vi "WF phase diversity_MATLAB_Correction_loop_AndorSDK_CorrForEachZ.vi"() -> ()   [LabVIEW 2018]
uses:
  <userlib>/WaveKit.lib/Controls/Wavefront Corrector states - ONE.ctl
  <userlib>/WaveKit.lib/Classes/WavefrontCorrector/WavefrontCorrector.lvclass
  <userlib>/WaveKit.lib/Classes/WavefrontCorrectorSet/WavefrontCorrectorSet.lvclass
  <vilib>/Analysis/1siggen.llb/Ramp Pattern by Samples.vi
  <vilib>/Utility/file.llb/Read From Spreadsheet File (DBL).vi
  <vilib>/Analysis/1siggen.llb/Ramp Pattern by Delta.vi
  <vilib>/Analysis/NI_AALBase.lvlib
panel:
  in  "Tab Control":T1(tab)
  in  "Offset command file":path=path "D:/SystemAlignment/system_aberration_20200206.dat"
  in  "Initial haso file":path=path "D:/SystemAlignment/system_aberration_residual_20191015.has"
  out "# of Phase":i32
  in  "Error in":errorcluster
  in  "DM configuration file":path=path "C:/Program Files (x86)/Imagine Optic/Configuration Files/WaveFrontCorrector_mirao52-e_0326.dat"
  out "DM Initial State":T2[](array[typedef])
  out "DM ActuatorsNumber":i32
  out "Error out":errorcluster
  in  "EMCCD trigger port":tag="Dev1/port0/line0"
  in  "Cooler set to Temperature":i32=-60
  in  "Trigger":u32(ring)=1 items=["Internal", "External"]
  out "Return from CheckTimings":u32
  out "Calculated Exposure Value":sgl format="%.2f"
  out "Return from SetTemperature":u32
  out "Cooling":i32
  out "Return from Initialize":u32
  out "Detector X Pixels":i32
  out "Detector Y Pixels":i32
  in  "Initialize EMCCD?":bool=TRUE
  in  "Turn off EMCCD when finished?":bool=TRUE
  in  "Initial Zer coeff":dbl[](array[numeric])=[0.2, 0.2]
  in  "Initial Zer index":dbl[](array[numeric])=[4.0, 5.0]
  out "Initial Zer coeff\nRandomly generated":dbl[](array[numeric])
  out "Initial Zer index (starting from 4)\nrandomly generated":dbl[](array[numeric])
  in  "aberration tolerance":dbl=0.1 format="%#_13g"
  in  "aberration threshold":dbl=0.25 format="%#_13g"
  in  "?":enum16{"input manually ", "randomly generated"}(ring)
  in  "max random order":i64=9
  in  "NOT YET: Data Acquisition Iteration #":i32=1
  in  "Zern index in 2":i32[](array[numeric])=[3, 4, 5, 6, 7, 8]
  in  "Zern coef in 2":sgl[](array[numeric])=[0.0, 0.0, 0.2, 0.0, 0.0, 0.0]
  in  "Zern index in 3":i32[](array[numeric])=[3, 4, 5, 6, 7, 8]
  in  "Zern coef in 3":sgl[](array[numeric])=[0.2, 0.0, 0.0, 0.0, 0.0, 0.0]
  in  "Zern index in 4":i32[](array[numeric])=[3, 4, 5, 6, 7, 8]
  in  "Zern coef in 4":sgl[](array[numeric])=[0.2, 0.0, 0.0, 0.0, 0.0, 0.0]
  in  "Zern index in 5":i32[](array[numeric])=[3, 4, 5, 6, 7, 8]
  in  "Zern coef in 5":sgl[](array[numeric])=[0.0, 0.0, 0.0, 0.0, 0.0, -0.2]
  in  "Andor Picture/notes save to path":path=path "D:/YD/test/test1"
  in  "base name":string="beads_test"
  in  "Pics/phase":dbl=2.0
  in  "camera exposure time (s)":string="0.02"
  in  "# of Phase":i32=5
  in  "COMMAND matrix path":path=path "D:/SystemAlignment/IM_20200224.aomi"
  in  "488 shutter":refnum<k7>(container)
  in  "?":bool
  out "phase diversity file name":string
  out "Corrected Picture name":string
  in  "Z scanning range (um)":dbl format="%#_13g"
  in  "Z scanning step (um)":dbl format="%#_13g"
  in  "center Z (um) (10 steps=1um)":dbl format="%#_13g"
  in  "ASI stage VISA resource name":refnum<visa-resource-name>="COM5"
  out "current z step (10 steps=1um)":string="where z"
  in  "Use GPU":bool=TRUE
  in  "Show Recon":bool=TRUE
  in  "Show Input":bool
  in  "Background Value":u32=290
  in  "Crop Size of image":u32=512
  in  "Gamma Value":dbl=1e-06
  in  "Iteration Number":u32=10
  in  "Zernike Order":u32=15
  in  "Number for average":u32=2
  in  "Number of Phase":u32=2
  in  "Run MATLAB or correction?":bool=TRUE
  in  "Keep Reconstructed Defocus component?":bool
  # "Cooler is off for testing"
  # "If Pics/phase is 2:\npicture order:\n\noffset+aberr *2\nphase diversity *8\n\nground truth *1\noffset+aberr *1\ncorrected *2 but the last one cannot be seen in imagej"
  # "Randomly Generate Initial Zernike, enter here:"
  # "Manually input, enter here:"
  # "Andor Camera Settings"
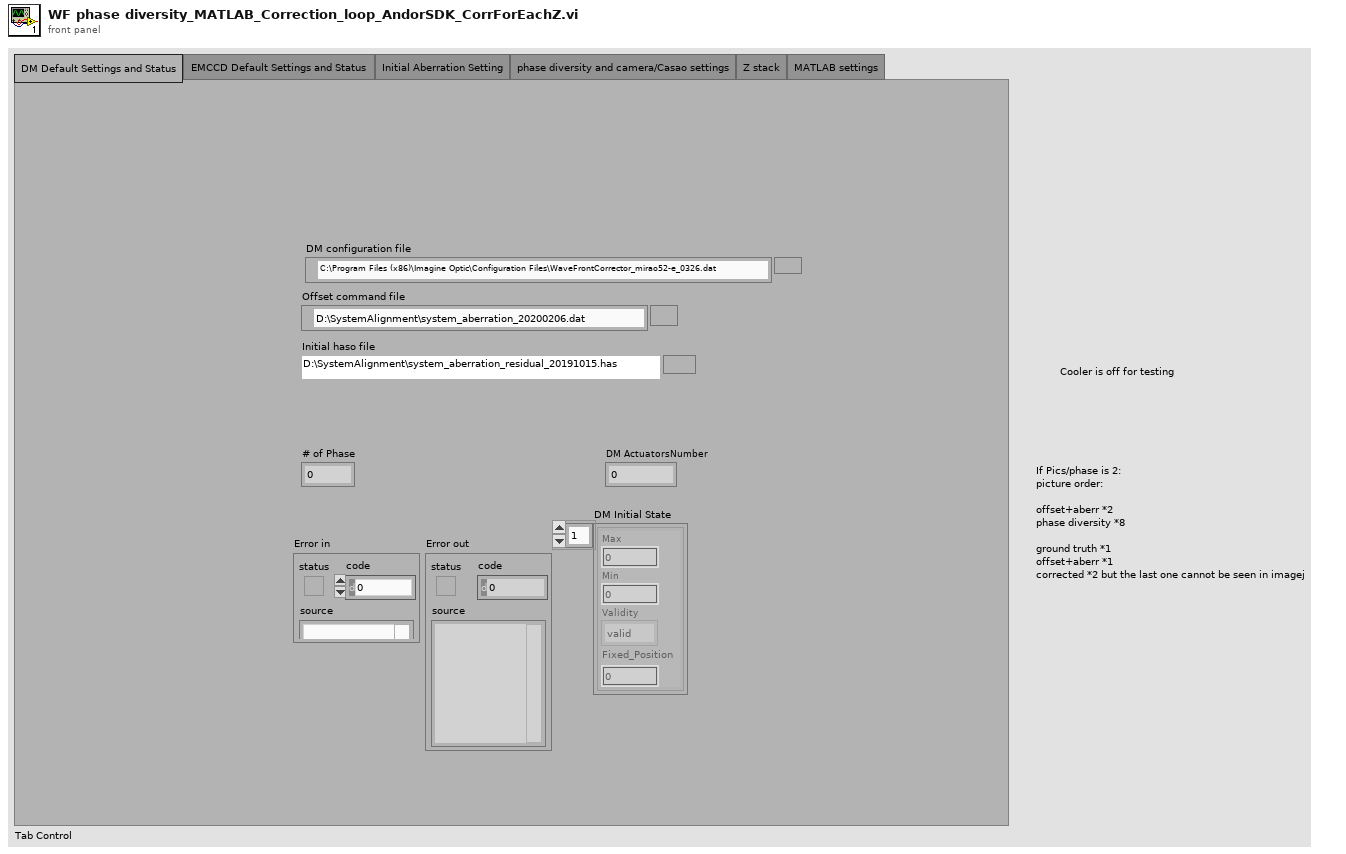
[diagram p1: front panel]
types:
  T1 = enum32{"DM Default Settings and Status", "EMCCD Default Settings and Status ", "Initial Aberration Setting", "phase diversity and camera/Casao settings", "Z stack", "MATLAB settings"}
  T2 = typedef "Wavefront Corrector states - ONE.ctl" = cluster{"Max":sgl, "Min":sgl, "Validity":enum16{"valid", "fixed", "invalid"}, "Fixed_Position":sgl}
  T3 = typedef "Error Code Enum typedef.ctl" = enum32{"N/A (0)", "DRV_ERROR_CODES", "DRV_SUCCESS", "DRV_VXDNOTINSTALLED", "DRV_ERROR_SCAN", "DRV_ERROR_CHECK_SUM", "DRV_ERROR_FILELOAD", "DRV_UNKNOWN_FUNC", "DRV_ERROR_VXD_INIT", "DRV_ERROR_ADDRESS", "DRV_ERROR_PAGELOCK", "DRV_ERROR_PAGEUNLOCK", "DRV_ERROR_BOARDTEST", "DRV_ERROR_ACK", "DRV_ERROR_UP_FIFO", "DRV_ERROR_PATTERN", "N/A (16)", "DRV_ACQUISITION_ERRORS", "DRV_ACQ_BUFFER", "DRV_ACQ_DOWNFIFO_FULL", "DRV_PROC_UNKONWN_INSTRUCTION", "DRV_ILLEGAL_OP_CODE", "DRV_KINETIC_TIME_NOT_MET", "DRV_ACCUM_TIME_NOT_MET", "DRV_NO_NEW_DATA", "N/A (25)", "DRV_SPOOLERROR", "N/A (27)", "N/A (28)", "N/A (29)", "N/A (30)", "N/A (31)", "N/A (32)", "DRV_TEMPERATURE_CODES", "DRV_TEMPERATURE_OFF", "DRV_TEMPERATURE_NOT_STABILIZED", "DRV_TEMPERATURE_STABILIZED", "DRV_TEMPERATURE_NOT_REACHED", "DRV_TEMPERATURE_OUT_RANGE", "DRV_TEMPERATURE_NOT_SUPPORTED", "DRV_TEMPERATURE_DRIFT", "N/A (41)", "N/A (42)", "N/A (43)", "N/A (44)", "N/A (45)", "N/A (46)", "N/A (47)", "N/A (48)", "DRV_GENERAL_ERRORS", "DRV_INVALID_AUX", "DRV_COF_NOTLOADED", "DRV_FPGAPROG", "DRV_FLEXERROR", "DRV_GPIBERROR", "N/A (55)", "N/A (56)", "N/A (57)", "N/A (58)", "N/A (59)", "N/A (60)", "N/A (61)", "N/A (62)", "N/A (63)", "DRV_DATATYPE", "DRV_DRIVER_ERRORS", "DRV_P1INVALID", "DRV_P2INVALID", "DRV_P3INVALID", "DRV_P4INVALID", "DRV_INIERROR", "DRV_COFERROR", "DRV_ACQUIRING", "DRV_IDLE", "DRV_TEMPCYCLE", "DRV_NOT_INITIALIZED", "DRV_P5INVALID", "DRV_P6INVALID", "DRV_INVALID_MODE", "DRV_INVALID_FILTER", "DRV_I2CERRORS", "DRV_I2CDEVNOTFOUND", "DRV_I2CTIMEOUT", "DRV_P7INVALID", "N/A (84)", "N/A (85)", "N/A (86)", "N/A (87)", "N/A (88)", "N/A (89)", "DRV_IOCERROR", "DRV_VRMVERSIONERROR"}
  T4 = typedef "NI_Matrix.lvlib/RealMatrix.ctl" = dbl[][]
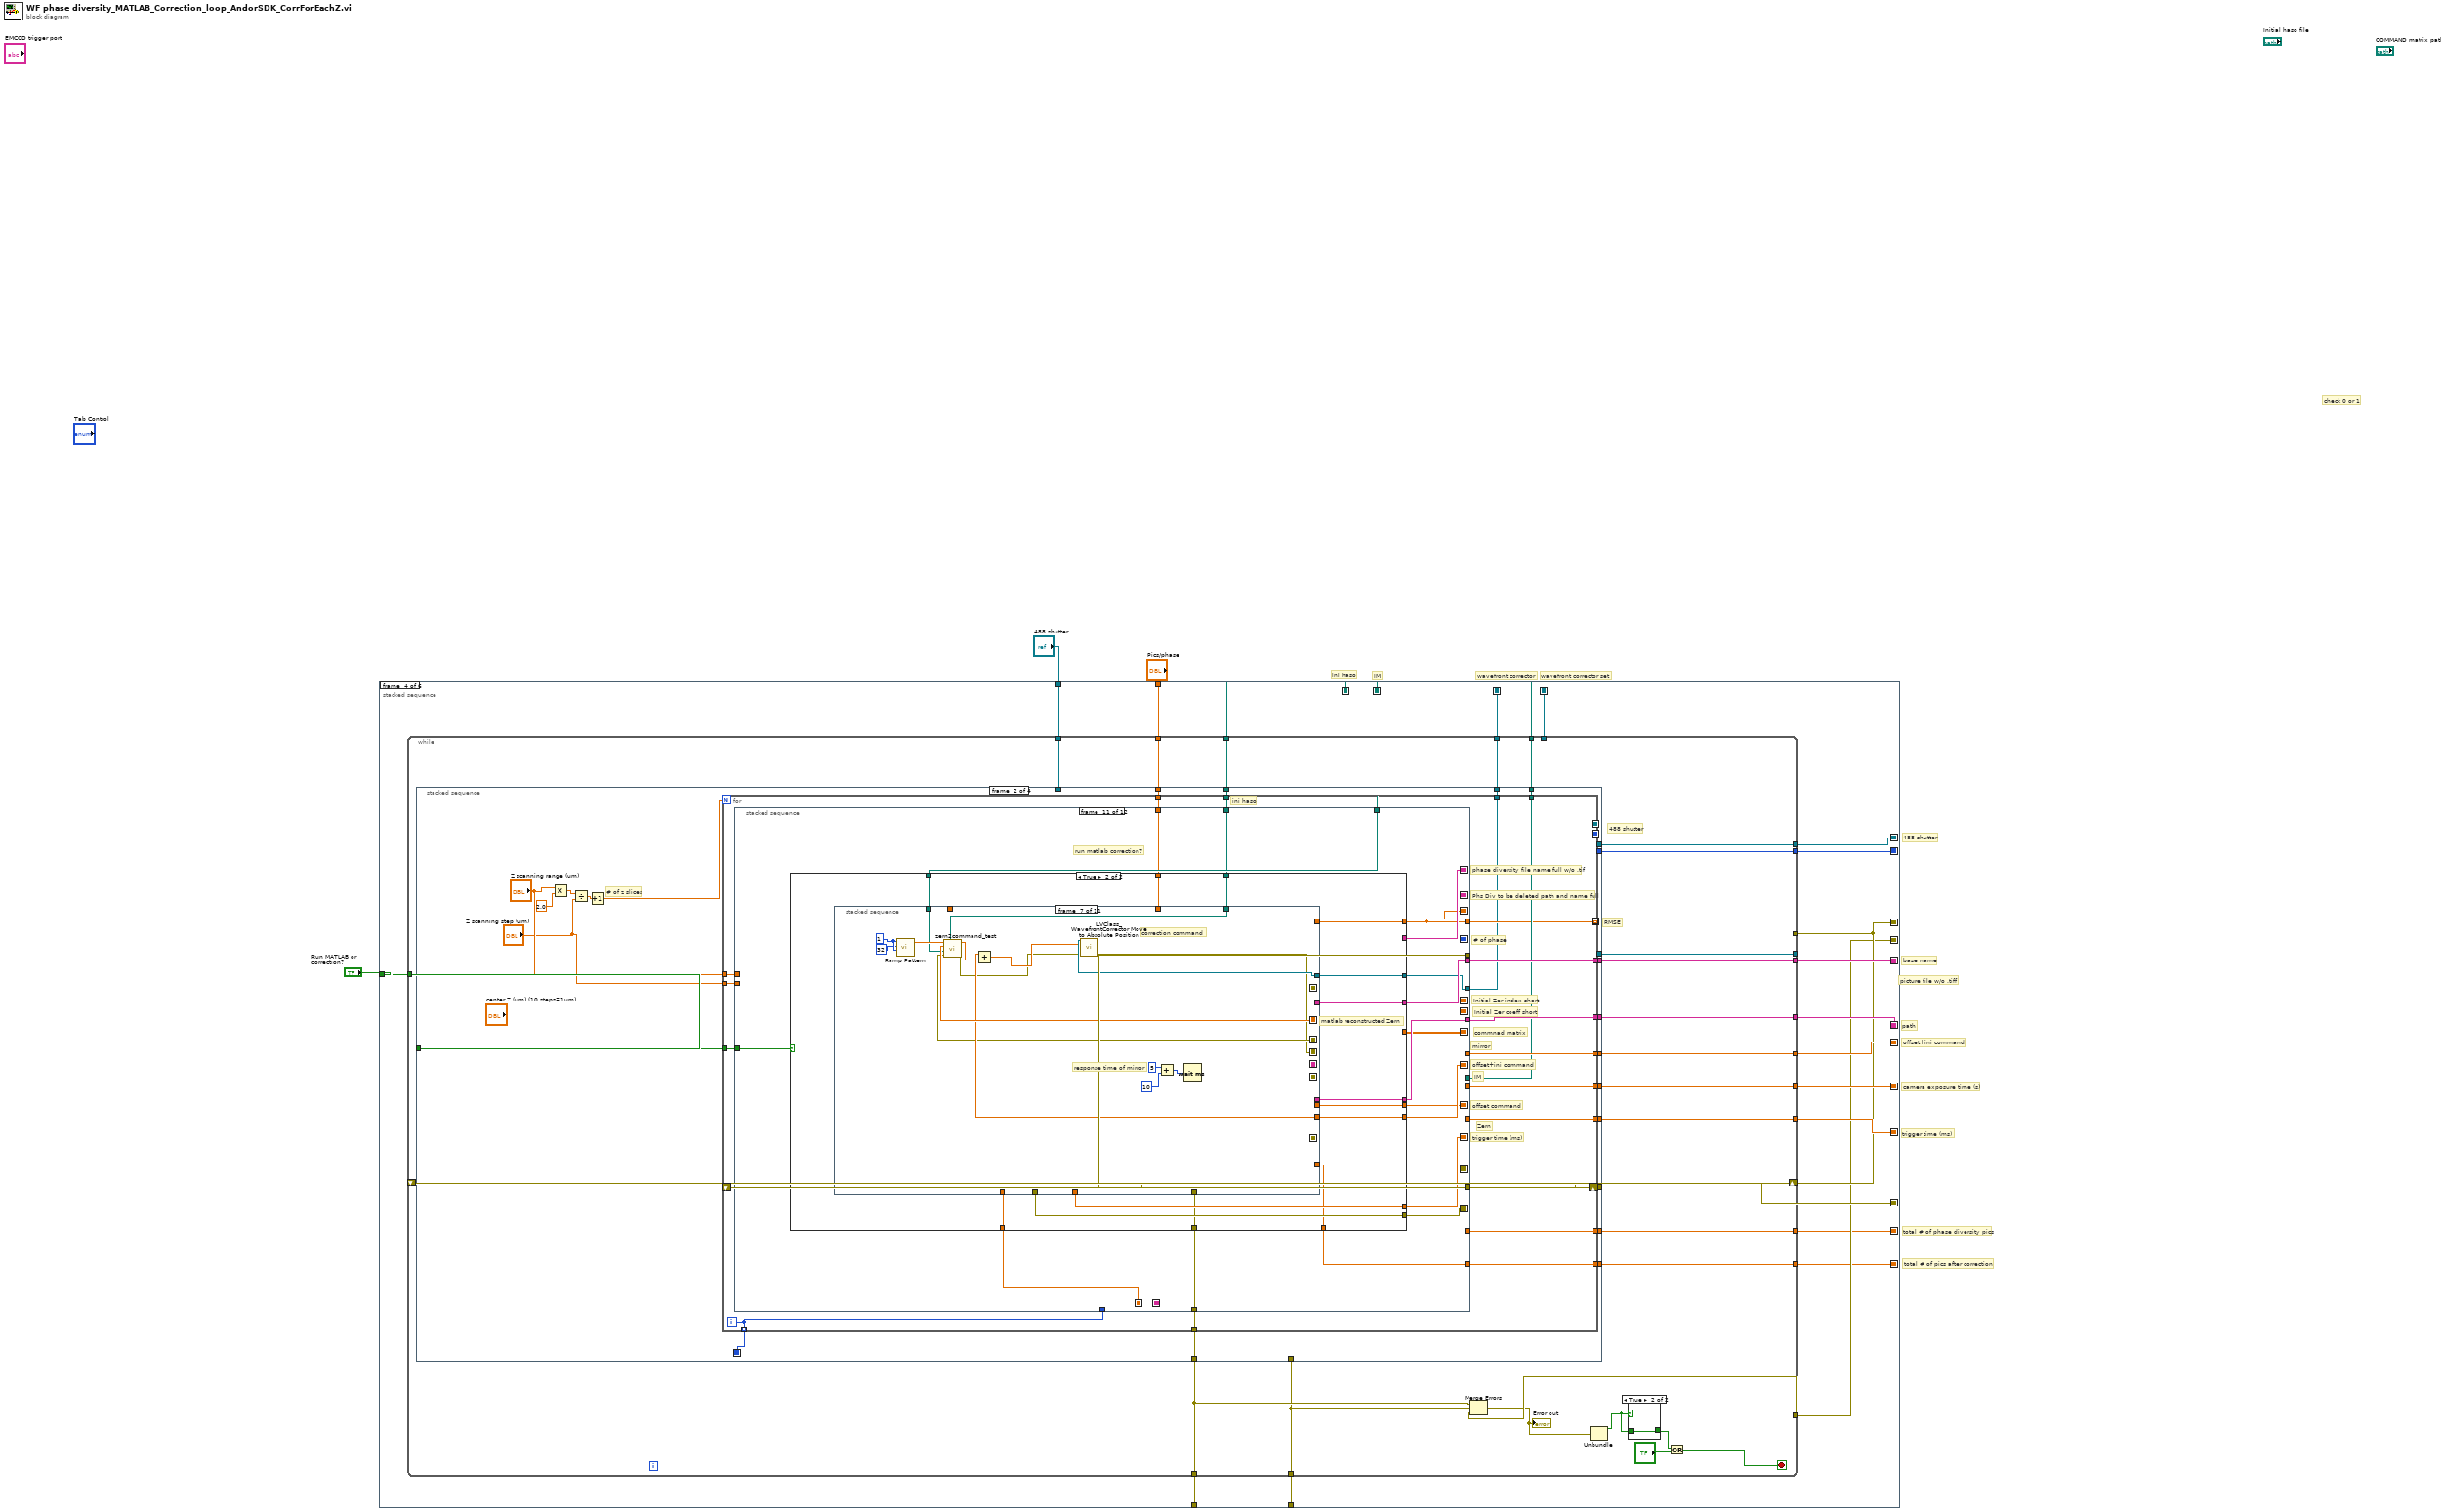
[diagram p0: block diagram]
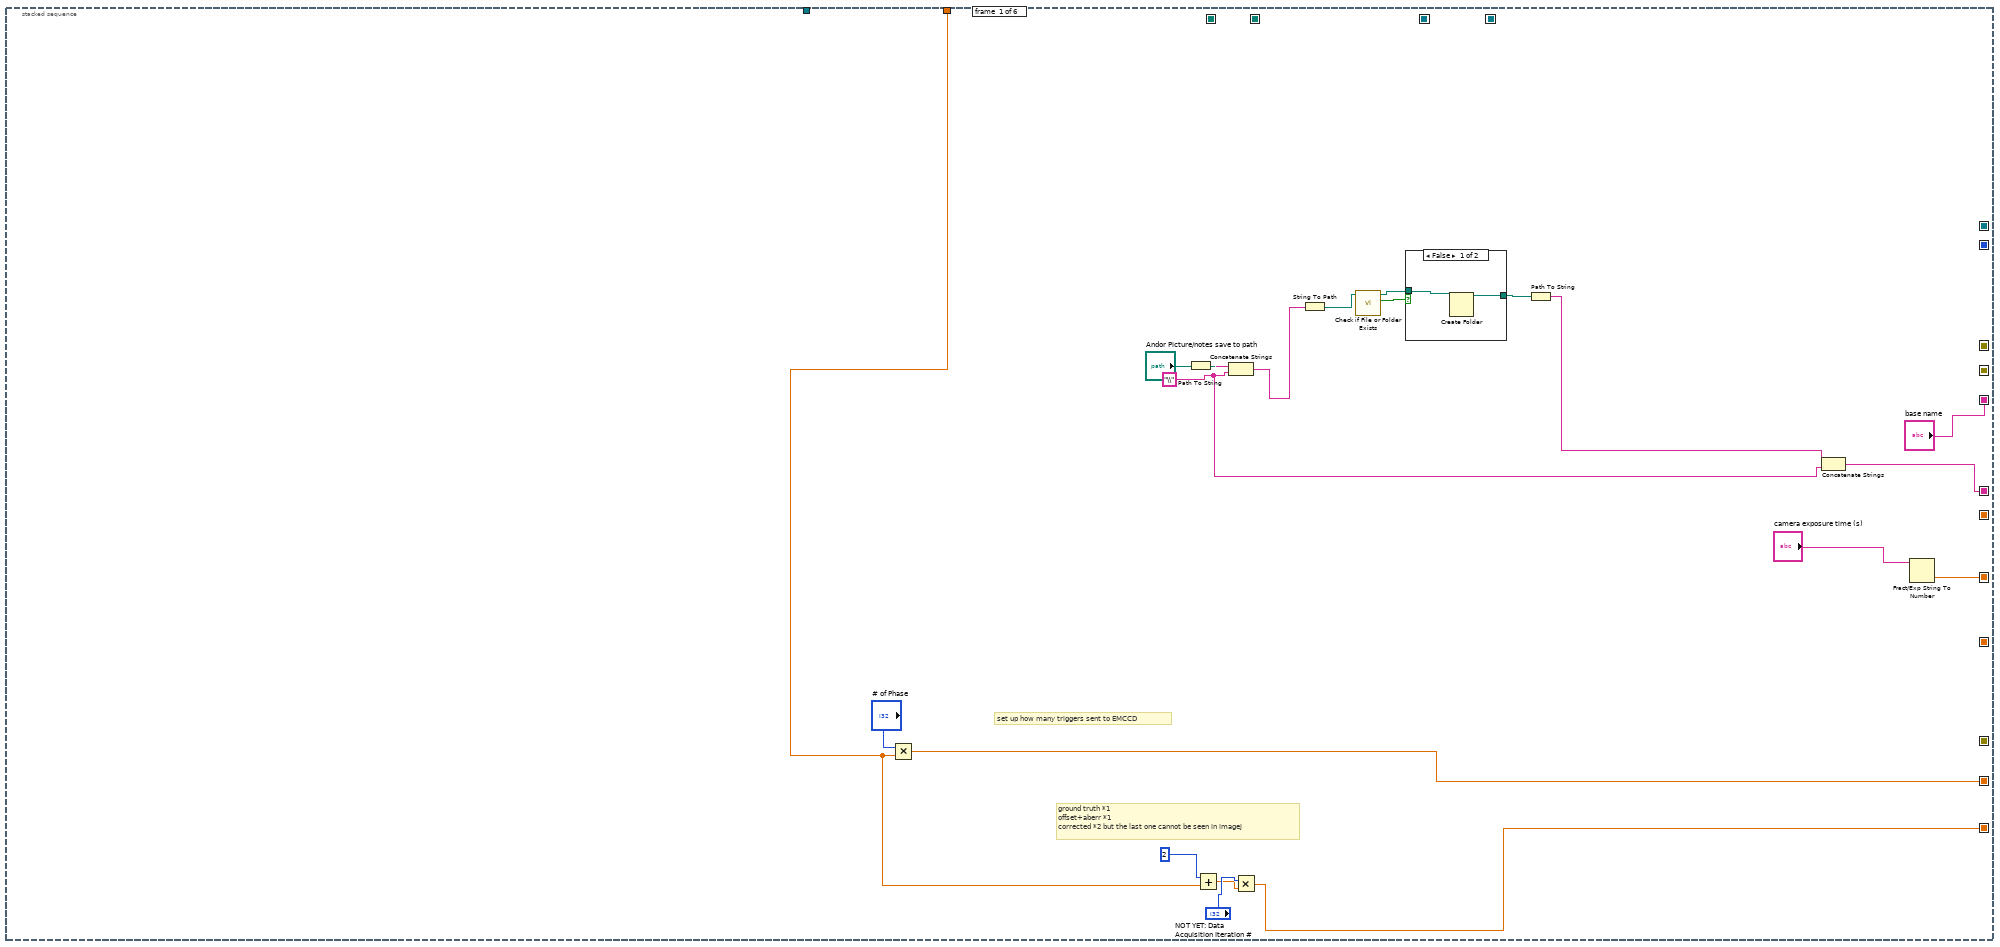
[diagram p2: hidden frame]
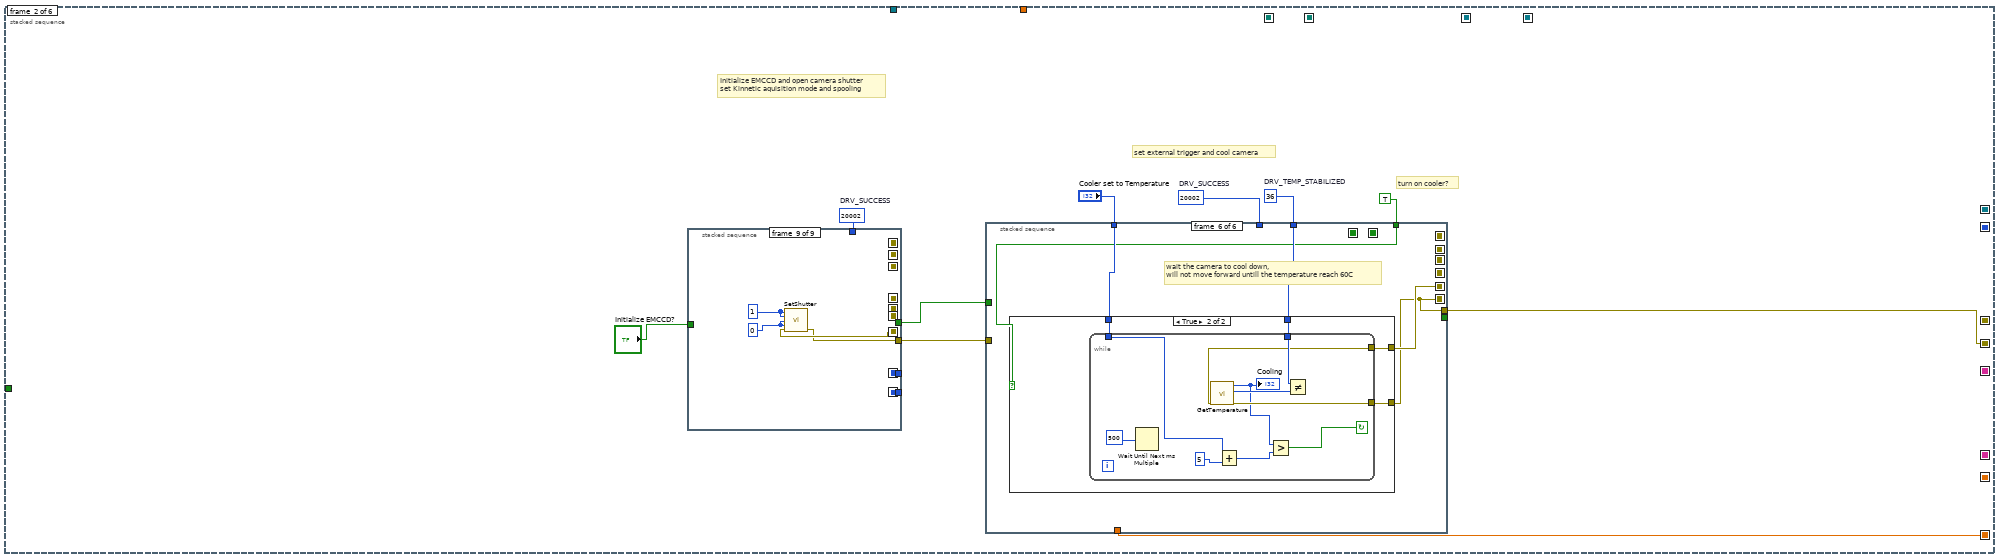
[diagram p4: hidden frame]
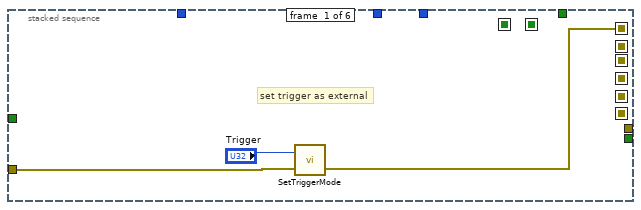
[diagram p5: hidden frame]
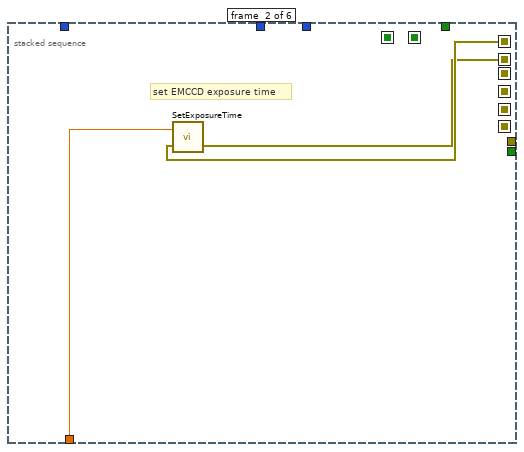
[diagram p6: hidden frame]
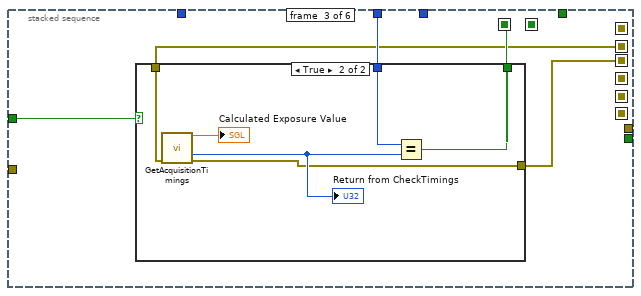
[diagram p7: hidden frame]
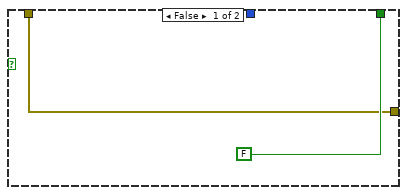
[diagram p8: hidden frame]
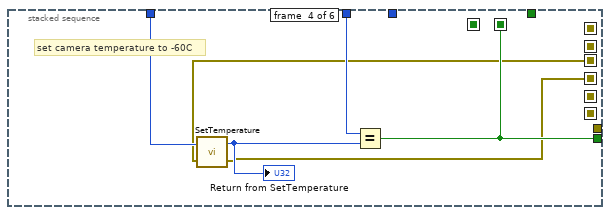
[diagram p9: hidden frame]
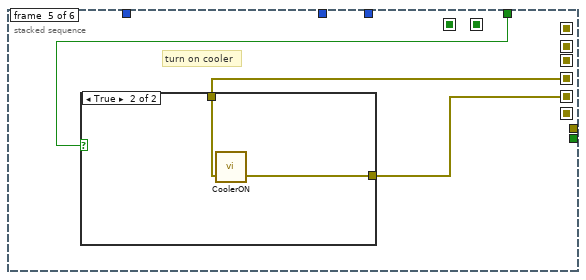
[diagram p10: hidden frame]
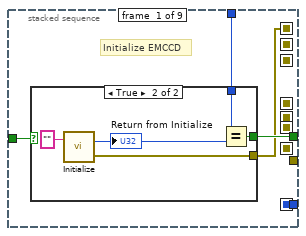
[diagram p13: hidden frame]
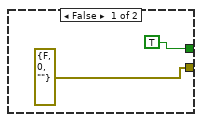
[diagram p14: hidden frame]
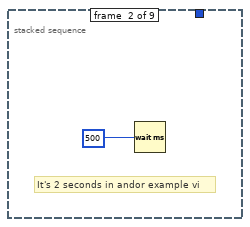
[diagram p15: hidden frame]
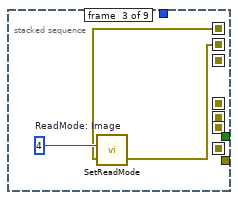
[diagram p16: hidden frame]
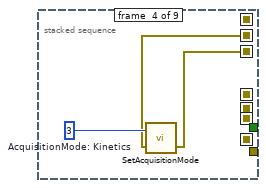
[diagram p17: hidden frame]
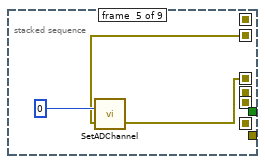
[diagram p18: hidden frame]
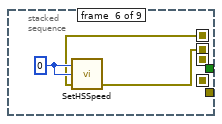
[diagram p19: hidden frame]
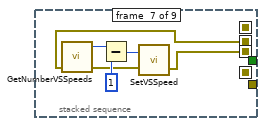
[diagram p20: hidden frame]
diagram:
  # "total # of phase diversity pics"
  # "picture file w/o .tiff"
  # "total # of pics after correction"
  # "wavefront corrector set"
  # "wavefront corrector"
  # "488 shutter"
  # "trigger time (ms)"
  # "offset+ini command"
  # "camera exposure time (s)"
  # "IM"
  # "ini haso"
  # "path"
  # "base name"
  # "check 0 or 1"
  n1 = stacked-sequence {
    seq-local: [w4 _ _ _ _ _] -> [_ _ _ w166 _ _]
    seq-local: ["base name" _ _ _ _ _] -> [_ _ _ w165 _ _]
    seq-local: [_ _ w146 _ _ _] -> [_ _ _ w164 _ _]
    seq-local: [_ _ w145 _ _ _] -> [_ _ _ w159 _ _]
    seq-local: [w18 _ _ _ _ _] -> [_ w29 _ w163 _ _]
    seq-local: [_ _ w130 _ _ _] -> [_ _ _ w151 _ _]
    seq-local: [_ _ _ w162 _ _] -> [_ _ _ _ _ _]
    seq-local: [_ _ _ w161 _ _] -> [_ _ _ _ _ _]
    seq-local: [_ _ _ w160 _ _] -> [_ _ _ _ _ w651]
    seq-local: [_ _ _ w154 _ _] -> [_ _ _ _ _ _]
    seq-local: [_ _ _ w157 _ _] -> [_ _ _ _ _ _]
    seq-local: [_ _ w129 _ _ _] -> [_ _ _ w152 _ w653]
    seq-local: [_ _ w128 _ _ _] -> [_ _ _ w150 _ w652]
    seq-local: [w15 _ _ _ _ _] -> [_ _ _ w147 _ _]
    seq-local: [_ w30 _ _ _ _] -> [_ _ _ w149 _ _]
    seq-local: [w14 _ _ _ _ _] -> [_ _ _ w148 _ _]
    tunnel: "Pics/phase" -> [w12 _ _ w167 _ _]
    tunnel: "Run MATLAB or correction?" -> [_ _ _ w158 _ _]
    tunnel: [_ _ _ w156 _ _] -> _
    tunnel: [_ _ _ w155 _ _] -> _
    tunnel: "488 shutter" -> [_ _ _ w153 _ w654]
    frame #0 {
      w5 = "\\"
      # "set up how many triggers sent to EMCCD"
      # "ground truth *1\noffset+aberr *1\ncorrected *2 but the last one cannot be seen in imagej"
      n2 = Multiply(x="# of Phase", y=w12) -> (x*y=w14:dbl)
      n3 = Path To String(path="Andor Picture/notes save to path") -> (string=w20:string)
      n4 = Add(x=2, y=w12) -> (x+y=w16:dbl)
      n5 = Concatenate Strings(w20, w5) -> (w7:string)
      n6 = Multiply(x="NOT YET: Data Acquisition Iteration #", y=w16) -> (x*y=w15:dbl)
      n7 = String To Path(string=w7) -> (path=w11:path)
      n8 = call <vilib>:"Check if File or Folder Exists.vi"("path"=w11) -> ("file or folder exists?"=w9:bool, "dup path"=w10:path)  [unwired: 8 in, 1 out]
      n9 = case shown="False" w9 {
        tunnel: w10 -> [w25 w26]
        tunnel: [w24 w26] -> w8
        frame False {
          n10 = Create Folder(path (use dialog)=w25) -> (created path=w24:path)  [unwired: 2 in, 2 out]
        }
        frame True {
        }
      }
      n11 = Path To String(path=w8) -> (string=w6:string)
      n12 = Concatenate Strings(w6, w5) -> (w4:string)
      n13 = Fract/Exp String To Number(string="camera exposure time (s)") -> (number=w18:dbl)  [unwired: 3 in, 1 out]
    }
    frame #1 {
      w32 = 36  # DRV_TEMP_STABILIZED
      w34 = 20002  # DRV_SUCCESS
      w36 = 20002  # DRV_SUCCESS
      # "turn on cooler?"
      # "set external trigger and cool camera"
      # "Initialize EMCCD and open camera shutter\nset Kinnetic aquisition mode and spooling"
      n14 = stacked-sequence {
        seq-local: [_ _ _ _ _ _ _ w122 _] -> [_ _ _ _ _ _ _ _ _]
        seq-local: [_ _ _ _ _ _ _ w121 _] -> [_ _ _ _ _ _ _ _ _]
        seq-local: [w89 _ _ _ _ _ _ _ _] -> [_ _ w101 _ _ _ _ _ _]
        seq-local: [_ _ w100 _ _ _ _ _ _] -> [_ _ _ w104 _ _ _ _ _]
        seq-local: [_ _ _ w103 _ _ _ _ _] -> [_ _ _ _ w106 _ _ _ _]
        seq-local: [_ _ _ _ w107 _ _ _ _] -> [_ _ _ _ _ w110 _ _ _]
        seq-local: [_ _ _ _ _ w109 _ _ _] -> [_ _ _ _ _ _ w114 _ _]
        seq-local: [_ _ _ _ _ _ w112 _ _] -> [_ _ _ _ _ _ _ w120 _]
        seq-local: [_ _ _ _ _ _ _ w118 _] -> [_ _ _ _ _ _ _ _ w125]
        tunnel: w36 -> [w91 _ _ _ _ _ _ _ _]
        tunnel: [w90 _ _ _ _ _ _ _ _] -> w35
        tunnel: [_ _ _ _ _ _ _ w122 _] -> _
        tunnel: [_ _ _ _ _ _ _ w121 _] -> _
        tunnel: [_ _ _ _ _ _ _ _ w124] -> w31
        tunnel: "Initialize EMCCD?" -> [w88 _ _ _ _ _ _ _ _]
        frame #0 {
          # "Initialize EMCCD"
          n15 = case shown="True" w88 {
            tunnel: w91 -> [_ w96]
            tunnel: [TRUE w95] -> w90
            tunnel: [errorcluster {"status"=FALSE, "code"=0, "source"=""} ("Error in 2") w94] -> w89
            frame False {
            }
            frame True {
              n16 = call <userlib>:"Initialize.vi"("directory (\"\")"="" ("directory (\"\")")) -> ("error out"=w94:errorcluster, "DLL error code"=w98:u32)  [unwired: 1 in]
              "Return from Initialize" <- w98
              n17 = Equal?(x=w96, y=w98) -> (x = y?=w95:bool)
            }
          }
        }
        frame #1 {
          # "It's 2 seconds in andor example vi"
          n18 = Wait (ms)(milliseconds to wait=u32 500) -> ()  [unwired: 1 out]
        }
        frame #2 {
          w102 = u16 4  # ReadMode: Image
          n19 = call <userlib>:"SetReadMode.vi"("error in (no error)"=w101, "mode"=w102) -> ("error out"=w100:errorcluster)  [unwired: 1 out]
        }
        frame #3 {
          w105 = u16 3  # AcquisitionMode: Kinetics
          n20 = call <userlib>:"SetAcquisitionMode.vi"("error in (no error)"=w104, "mode"=w105) -> ("error out"=w103:errorcluster)  [unwired: 1 out]
        }
        frame #4 {
          n21 = call <userlib>:"SetADChannel.vi"("error in (no error)"=w106, "channel"=0) -> ("error out"=w107:errorcluster)  [unwired: 1 out]
        }
        frame #5 {
          w111 = 0
          n22 = call <userlib>:"SetHSSpeed.vi"("error in (no error)"=w110, "index"=w111, "type"=w111) -> ("error out"=w109:errorcluster)  [unwired: 1 in, 1 out]
        }
        frame #6 {
          n23 = call <userlib>:"GetNumberVSSpeeds.vi"("error in (no error)"=w114) -> ("error out"=w113:errorcluster, "number"=w117:i32)  [unwired: 2 in, 1 out]
          n24 = Subtract(x=w117, y=1) -> (x-y=w115:i32)
          n25 = call <userlib>:"SetVSSpeed.vi"("error in (no error)"=w113, "index"=w115) -> ("error out"=w112:errorcluster)  [unwired: 1 out]
        }
        frame #7 {
          w123 = 1
          n26 = call <userlib>:"GetDetector.vi"("error in (no error)"=w120) -> ("error out"=w119:errorcluster, "ypixels"=w122:i32, "xpixels"=w121:i32)  [unwired: 3 in, 1 out]
          "Detector Y Pixels" <- w122
          "Detector X Pixels" <- w121
          n27 = call <userlib>:"SetImage.vi"("hbin"=w123, "vbin"=w123, "hstart"=w123, "hend"=w121, "vstart"=w123, "vend"=w122, "error in (no error)"=w119) -> ("error out"=w118:errorcluster)  [unwired: 19 in, 1 out]
        }
        frame #8 {
          w126 = 0
          w127 = 1
          n28 = call <userlib>:"SetShutter.vi"("type"=w127, "mode"=w127, "closingtime"=w126, "openingtime"=w126, "error in (no error)"=w125) -> ("error out"=w124:errorcluster)  [unwired: 9 in, 1 out]
        }
      }
      n29 = stacked-sequence {
        seq-local: [_ _ w45 _ _ _] -> [_ _ _ _ _ _]
        seq-local: [_ _ _ w58 _ _] -> [_ _ _ _ _ _]
        seq-local: [w37 _ _ _ _ _] -> [_ w42 _ _ _ _]
        seq-local: [_ w41 _ _ _ _] -> [_ _ w44 _ _ _]
        seq-local: [_ _ w43 _ _ _] -> [_ _ _ w57 _ _]
        seq-local: [_ _ _ w56 _ _] -> [_ _ _ _ w64 _]
        seq-local: [_ _ _ _ w63 _] -> [_ _ _ _ _ w70]
        seq-local: [_ _ _ _ _ w68] -> [_ _ _ _ _ _]
        tunnel: w34 -> [_ _ w47 w61 _ _]
        tunnel: "Cooler set to Temperature" -> [_ _ _ w59 _ w71]
        tunnel: w32 -> [_ _ _ _ _ w72]
        tunnel: [_ _ _ w58 _ _] -> _
        tunnel: w35 -> [_ _ w46 _ _ _]
        tunnel: w31 -> [w38 _ _ _ _ _]
        tunnel: [_ _ _ _ _ w68] -> w30
        tunnel: w29 -> [_ w40 _ _ _ _]
        tunnel: TRUE -> [_ _ _ _ w62 w69]
        frame #0 {
          # "set trigger as external"
          n30 = call <userlib>:"SetTriggerMode.vi"("error in (no error)"=w38, "mode"="Trigger") -> ("error out"=w37:errorcluster)  [unwired: 1 out]
        }
        frame #1 {
          # "set EMCCD exposure time"
          n31 = call <userlib>:"SetExposureTime.vi"("error in (no error)"=w42, "time"=w40) -> ("error out"=w41:errorcluster)  [unwired: 1 out]
        }
        frame #2 {
          n32 = case shown="True" w46 {
            tunnel: w47 -> [_ w53]
            tunnel: [FALSE w55] -> w45
            tunnel: w44 -> [w48 w51]
            tunnel: [w48 w50] -> w43
            frame False {
            }
            frame True {
              n33 = call <userlib>:"GetAcquisitionTimings.vi"("error in (no error)"=w51) -> ("exposure"=→"Calculated Exposure Value":sgl, "DLL error code"=w52:u32, "error out"=w50:errorcluster)  [unwired: 10 in, 2 out]
              "Return from CheckTimings" <- w52
              n34 = Equal?(x=w53, y=w52) -> (x = y?=w55:bool)
            }
          }
        }
        frame #3 {
          # "set camera temperature to -60C"
          n35 = call <userlib>:"SetTemperature.vi"("error in (no error)"=w57, "temperature"=w59) -> ("error out"=w56:errorcluster, "DLL error code"=w60:u32)
          "Return from SetTemperature" <- w60
          n36 = Equal?(x=w61, y=w60) -> (x = y?=w58:bool)
        }
        frame #4 {
          # "turn on cooler"
          n37 = case shown="True" w62 {
            tunnel: w64 -> [w65 w67]
            tunnel: [w65 w66] -> w63
            frame False {
            }
            frame True {
              n38 = call <userlib>:"CoolerON.vi"("error in (no error)"=w67) -> ("error out"=w66:errorcluster)  [unwired: 1 in, 1 out]
            }
          }
        }
        frame #5 {
          # "wait the camera to cool down,\nwill not move forward untill the temperature reach 60C"
          n39 = case shown="True" w69 {
            tunnel: w72 -> [_ w77]
            tunnel: w71 -> [_ w76]
            tunnel: w70 -> [w73 w75]
            tunnel: [w73 w74] -> w68
            frame False {
            }
            frame True {
              n40 = while {
                tunnel: w77 -> [w86]
                tunnel: w76 -> [w79]
                tunnel: w75 -> [w84]
                tunnel: [w83] -> w74
                stop <- w78 continue-if-true
                n41 = Wait Until Next ms Multiple(millisecond multiple=u32 500) -> ()  [unwired: 1 out]
                n42 = call <userlib>:"GetTemperature.vi"("error in (no error)"=w84) -> ("error out"=w83:errorcluster, "status"=w85:T3, "temperature"=w80:i32)  [unwired: 3 in, 1 out]
                "Cooling" <- w80
                n43 = Add(x=w79, y=5) -> (x+y=w81:i32)
                n44 = Greater?(x=w80, y=w81) -> (0:w78:bool)
                n45 = Not Equal?(x=w86, y=w85) -> ()  [unwired: 1 out]
              }
            }
          }
        }
      }
    }
    frame #2 {
      # "Initialize CASAO"
      n46 = call <userlib>:"LVClass_WavefrontCorrectorSet ctor.vi"("WavefrontCorrectorSet in"=refnum<class "WavefrontCorrectorSet.lvclass"> refnum, "PathToWavefrontCorrectorSetupFile"="DM configuration file", "error in (no error)"="Error in") -> ("WavefrontCorrectorSet out"=w135:refnum<class "WavefrontCorrectorSet.lvclass">, "error out"=w144:errorcluster)  [unwired: 11 in]
      n47 = call <userlib>:"LVClass_WavefrontCorrector ctor.vi"("WavefrontCorrector in"=refnum<class "WavefrontCorrector.lvclass"> refnum, "PathToWavefrontCorrectorSetupFile"="DM configuration file", "error in (no error)"=w144) -> ("WavefrontCorrector out"=w139:refnum<class "WavefrontCorrector.lvclass">, "error out"=w138:errorcluster)  [unwired: 11 in]
      n48 = call <userlib>:"LVClass_WavefrontCorrector Init.vi"("WavefrontCorrector in"=w139, "set_init_state_from_config_file"=TRUE, "error in (no error)"=w138) -> ("WavefrontCorrector out"=w133:refnum<class "WavefrontCorrector.lvclass">, "error out"=w137:errorcluster)  [unwired: 11 in]
      n49 = call <userlib>:"LVClass_WavefrontCorrectorSet get nb of actuators.vi"("WavefrontCorrectorSet in"=w135, "error in (no error)"=w137) -> ("WavefrontCorrectorSet out"=w128:refnum<class "WavefrontCorrectorSet.lvclass">, "ActuatorsNumber"=→"DM ActuatorsNumber":i32, "error out"=w134:errorcluster)  [unwired: 11 in]
      n50 = call <userlib>:"LVClass_WavefrontCorrector Get Current Preferences.vi"("WavefrontCorrector in"=w133, "error in (no error)"=w134) -> ("WavefrontCorrector out"=w129:refnum<class "WavefrontCorrector.lvclass">, "Mirror preferences.Wavefront Corrector State"=→"DM Initial State":T2[], "error out"=w130:errorcluster)  [unwired: 10 in, 1 out]
      n51 = local read "COMMAND matrix path"() -> (w145:path)
      n52 = local read "Initial haso file"() -> (w146:path)
    }
    frame #3 {
      n53 = while {
        tunnel: w167 -> [w193]
        tunnel: w166 -> [w192]
        tunnel: w165 -> [w191]
        tunnel: w164 -> [w190]
        tunnel: w163 -> [w189]
        tunnel: [w187] -> w162
        tunnel: [w186] -> w161
        tunnel: w159 -> [w184]
        tunnel: w158 -> [w183]
        tunnel: [w182] -> w157
        tunnel: [w181] -> _
        tunnel: [w179] -> w156
        tunnel: [w180] -> w155
        shift-right: [w185] -> w160
        shift-left: w151 -> [w188]
        tunnel: [w178] -> w154
        tunnel: w153 -> [w177]
        tunnel: w152 -> [w176]
        tunnel: w151 -> [_]
        tunnel: w150 -> [_]
        tunnel: w149 -> [w175]
        tunnel: w148 -> [w169]
        tunnel: w147 -> [w168]
        stop <- w171 stop-if-true
        # "488 shutter"
        # "RMSE"
        n54 = stacked-sequence {
          seq-local: [_ w215 _ _] -> [_ _ _ w644]
          seq-local: [_ w214 _ _] -> [_ _ _ _]
          seq-local: [w198 _ _ _] -> [_ _ w640 _]
          seq-local: [w199 _ _ _] -> [_ _ w639 _]
          tunnel: w193 -> [_ w226 _ _]
          tunnel: w192 -> [_ w225 _ w642]
          tunnel: w191 -> [_ w224 _ w641]
          tunnel: w190 -> [_ w223 _ _]
          tunnel: w189 -> [_ w222 _ _]
          tunnel: w188 -> [_ w221 _ _]
          tunnel: [_ w220 _ _] -> w187
          tunnel: [_ w219 _ _] -> w186
          tunnel: [_ w218 _ _] -> w185
          tunnel: w184 -> [_ w217 _ _]
          tunnel: w183 -> [_ w216 _ _]
          tunnel: [_ _ w638 _] -> w181
          tunnel: [_ _ w637 _] -> w182
          tunnel: [_ _ _ w643] -> w179
          tunnel: [_ w213 _ _] -> w180
          tunnel: [w198 _ _ _] -> w178
          tunnel: w177 -> [w197 _ _ _]
          tunnel: w176 -> [_ w212 _ _]
          tunnel: w169 -> [_ w211 _ _]
          tunnel: w168 -> [_ w210 _ _]
          frame #0 {
            # "open the shutter of 488nm laser"
            n55 = property class="MG17Motor"(reference=w197, "HWSerialNum"=85819115.0) -> (reference out=w203:refnum<k7>)  [unwired: 1 in, 1 out]
            n56 = invoke class="MG17Motor" method="StartCtrl"(reference=w203) -> (reference out=w201:refnum<k7>)  [unwired: 2 in, 2 out]
            n57 = invoke class="MG17Motor" method="SC_Enable"(reference=w201, "lChanID"=0) -> (reference out=w198:refnum<k7>, "lChanID"=w199:i32)  [unwired: 2 in, 2 out]
          }
          frame #1 {
            # "# of z slices"
            n58 = Multiply(x="Z scanning range (um)", y=2.0) -> (x*y=w208:dbl)
            n59 = Divide(x=w208, y="Z scanning step (um)") -> (x/y=w207:dbl)
            n60 = Increment(x=w207) -> (x+1=w206:dbl)
            n61 = for {
              N: w206 -> [_]
              tunnel: w226 -> [w245]
              tunnel: w225 -> [w244]
              tunnel: w224 -> [w243]
              tunnel: w223 -> [w242]
              tunnel: w222 -> [w241]
              tunnel: [w239] -> w220
              tunnel: [w238] -> w219
              tunnel: w217 -> [w236]
              tunnel: w216 -> [w235]
              shift-right: [w237] -> w218
              shift-left: w221 -> [w240]
              tunnel: [w234] -> w215 mode=indexing
              tunnel: [w233] -> w214 mode=indexing
              tunnel: [w232] -> w213
              tunnel: w212 -> [w231]
              tunnel: w211 -> [w230]
              tunnel: w210 -> [w229]
              tunnel: "Z scanning range (um)" -> [w228]
              tunnel: "Z scanning step (um)" -> [w227]
              i -> [w233]
              # "Phs Div to be deleted path and name full"
              # "phase diversity file name full w/o .tif"
              # "# of phase"
              # "trigger time (ms)"
              # "offset+ini command"
              # "Initial Zer coeff short"
              # "Initial Zer index short"
              # "mirror"
              # "Zern"
              # "commnad matrix"
              # "ini haso"
              # "IM"
              # "offset command"
              n62 = stacked-sequence {
                seq-local: [_ _ _ _ w276 _ _ _ _ _ _ _] -> [_ _ _ _ _ w296 _ w424 _ _ w480 _]
                seq-local: [_ _ _ _ _ w294 _ _ _ _ _ _] -> [_ _ _ _ _ _ _ w423 _ _ w481 _]
                seq-local: [_ _ _ _ _ w292 _ _ _ _ _ _] -> [_ _ _ _ _ _ _ w422 _ _ _ _]
                seq-local: [_ _ _ _ _ w285 _ _ _ _ _ _] -> [_ _ _ _ _ _ _ w419 _ _ _ _]
                seq-local: [_ _ _ w267 _ _ _ _ _ _ _ _] -> [_ _ _ _ _ w282 _ _ _ _ _ _]
                seq-local: [_ _ _ w266 _ _ _ _ _ _ _ _] -> [_ _ _ _ _ w281 _ _ _ _ _ _]
                seq-local: [_ _ _ _ _ w280 _ _ _ _ _ _] -> [_ _ _ _ _ _ _ _ _ _ w486 _]
                seq-local: [_ _ _ _ _ _ _ w418 _ _ _ _] -> [_ _ _ _ _ _ _ _ w459 _ w484 _]
                seq-local: [_ _ _ _ _ _ _ w417 _ _ _ _] -> [_ _ _ _ _ _ _ _ _ _ w483 _]
                seq-local: [_ _ _ _ _ _ _ _ _ w463 _ _] -> [_ _ _ _ _ _ _ _ _ _ w476 _]
                seq-local: [_ _ _ _ _ _ w411 _ _ _ _ _] -> [_ _ _ _ _ _ _ _ _ _ _ w618]
                seq-local: [w247 _ _ _ _ _ _ _ _ _ _ _] -> [_ _ _ _ _ w279 w408 _ _ w461 w475 _]
                seq-local: [w246 _ _ _ _ _ _ _ _ _ _ _] -> [_ _ _ _ _ _ _ _ _ _ _ _]
                seq-local: [_ _ _ _ _ _ _ _ _ _ w474 _] -> [_ _ _ _ _ _ _ _ _ _ _ _]
                tunnel: w245 -> [_ _ _ _ _ w289 _ w427 _ _ w485 _]
                tunnel: w244 -> [_ _ _ _ _ w290 w414 w426 _ w471 w488 _]
                tunnel: w243 -> [_ _ _ _ _ w291 w413 w425 _ w472 w489 _]
                tunnel: w242 -> [_ _ _ _ _ w288 _ _ _ _ w473 _]
                tunnel: w236 -> [_ _ _ _ _ w287 _ w421 _ _ _ _]
                tunnel: w241 -> [_ _ _ _ _ _ _ w420 _ _ _ _]
                tunnel: w240 -> [_ _ _ _ _ w286 _ _ _ _ _ _]
                tunnel: [_ _ _ _ _ _ _ w417 _ _ _ _] -> w237
                tunnel: [_ _ _ _ _ w280 _ _ _ _ _ _] -> w239
                tunnel: [_ _ _ _ _ _ _ w418 _ _ _ _] -> w238
                tunnel: w236 -> [_ _ _ _ _ _ _ _ _ _ w487 _]
                tunnel: w235 -> [_ _ _ _ _ _ _ _ _ _ w482 _]
                tunnel: w233 -> [w249 _ _ _ _ _ _ _ _ _ _ _]
                tunnel: [_ _ _ _ _ _ _ _ _ _ w474 _] -> w234
                tunnel: [_ _ _ _ _ _ _ _ _ _ w479 _] -> w232
                tunnel: w231 -> [_ _ _ _ _ _ _ w416 _ _ w478 _]
                tunnel: w230 -> [_ _ _ _ _ _ w415 _ _ _ _ w616]
                tunnel: w229 -> [_ _ _ _ _ _ _ _ _ _ w477 _]
                tunnel: w228 -> [w250 _ _ _ _ _ _ _ _ _ _ _]
                tunnel: w227 -> [w248 _ _ _ _ _ _ _ _ _ _ _]
                frame #0 {
                  # "10 step=1um"
                  # "move to z"
                  # "move to Z"
                  n63 = local read "center Z (um) (10 steps=1um)"() -> (w255:dbl)
                  n64 = local read "ASI stage VISA resource name"() -> (w256:refnum<visa-resource-name>)
                  n65 = Subtract(x=w255, y=w250) -> (x-y=w254:dbl)
                  n66 = Multiply(x=w248, y=w249) -> (x*y=w253:dbl)
                  n67 = Add(x=w254, y=w253) -> (x+y=w252:dbl)
                  n68 = Multiply(x=w252, y=10) -> (x*y=w247:dbl)
                  n69 = Number To Decimal String(number=w247) -> (decimal integer string=w246:string)  [unwired: 1 in]
                  n70 = Concatenate Strings("move z=", w246) -> (w257:string)
                  n71 = call "WriteCmd.vi"("Command"=w257, "VISA resource name"=w256) -> ()  [unwired: 1 in, 1 out]
                }
                frame #1 {
                  n72 = Wait (ms)(milliseconds to wait=300) -> ()  [unwired: 1 out]
                }
                frame #2 {
                  # "read z coordinate"
                  n73 = local read "ASI stage VISA resource name"() -> (w264:refnum<visa-resource-name>)
                  n74 = call "WriteCmd.vi"("Command"="where z", "VISA resource name"=w264) -> ("error"=w263:errorcluster)  [unwired: 1 in]
                  n75 = VISA Read(VISA resource name=w264, byte count=100 ("read count"), error in (no error)=w263) -> (read buffer=→"current z step (10 steps=1um)":string)  [unwired: 3 out]
                }
                frame #3 {
                  # "generate initial aberration (aberr to correct)"
                  n76 = case shown="\"randomly generated\"" "?" {
                    tunnel: ["Initial Zer index" w273] -> w267
                    tunnel: ["Initial Zer coeff" w272] -> w266
                    tunnel: "max random order" -> [_ w271]
                    frame "input manually " {
                    }
                    frame "randomly generated" {
                      # "generate random zernike index and coefficient arrays"
                      n77 = call "Random Aberration Array Generator.vi"("max random order"=w271, "aberration tolerance"="aberration tolerance", "aberration threshold"="aberration threshold") -> ("Zer coeff"=w272:dbl[], "Zer index (starting from 3)"=w273:dbl[])  [unwired: 7 in]
                      "Initial Zer index (starting from 4)\nrandomly generated" <- w273
                      "Initial Zer coeff\nRandomly generated" <- w272
                    }
                  }
                }
                frame #4 {
                  # "read in offset command"
                  n78 = call-poly <vilib>:"Read From Spreadsheet File.vi"("format (%.3f)"="%.8f", "file path (dialog if empty)"="Offset command file") -> ("first row"=w276:dbl[])  [unwired: 5 in, 4 out]
                }
                frame #5 {
                  w301 = 0.0
                  # "ini zern coeff"
                  # "offset+ini command"
                  # "Zern coeff"
                  # "Zern index"
                  # "calculate the command:\nfor phase diversity"
                  n79 = Array Size(array="Zern index in 2") -> (size(s)=w299:i32)
                  n80 = call-poly <vilib>:"Ramp Pattern.vi"("start"=w301, "end"=w301, "samples"=w299) -> ("Ramp Pattern"=w298:dbl[])  [unwired: 7 in, 1 out]
                  n81 = Build Array(w298, "Zern index in 2", "Zern index in 3", "Zern index in 4", "Zern index in 5") -> (w283:T4)
                  n82 = Build Array(w298, "Zern coef in 2", "Zern coef in 3", "Zern coef in 4", "Zern coef in 5") -> (w302:T4)
                  n83 = Transpose Matrix(1:w302) -> (0:w295:T4)
                  n84 = Transpose Matrix(1:w283) -> (0:w293:T4)
                  n85 = Array Size(array=w283) -> (size(s)=w284:i32[])
                  n86 = Index Array(array=w284, index=1) -> (element=w292:i32)
                  "# of Phase" <- w292
                  n87 = stacked-sequence {
                    seq-local: [w311 _ _] -> [_ w329 w395]
                    seq-local: [w312 _ _] -> [_ w323 _]
                    seq-local: [_ w322 _] -> [_ _ w392]
                    seq-local: [w310 _ _] -> [_ w321 _]
                    tunnel: w292 -> [_ w334 _]
                    tunnel: w282 -> [w319 _ _]
                    tunnel: w281 -> [w318 w324 _]
                    tunnel: w287 -> [w317 w331 _]
                    tunnel: w296 -> [w315 _ _]
                    tunnel: w293 -> [_ w333 _]
                    tunnel: w295 -> [_ w332 _]
                    tunnel: w288 -> [w314 w330 _]
                    tunnel: [_ w328 _] -> w294
                    tunnel: w291 -> [_ w326 w393]
                    tunnel: w290 -> [_ w327 w394]
                    tunnel: w289 -> [_ w325 _]
                    tunnel: w286 -> [w313 _ _]
                    tunnel: [_ _ w391] -> w285
                    tunnel: [w311 _ _] -> w280
                    tunnel: w279 -> [_ w320 w389]
                    frame #0 {
                      n88 = call "zern2command_test.vi"("Initial haso file"=w314, "error in (no error)"=w313, "interaction matrix file"=w317, "Zern coef in"=w318, "Zern index in"=w319) -> ("error out"=w312:errorcluster, "Zern coef out"=w310:sgl[], "Offset positions"=w316:sgl[])  [unwired: 4 in]
                      n89 = Add(x=w316, y=w315) -> (x+y=w311:dbl[])
                    }
                    frame #1 {
                      n90 = for {
                        N: w334 -> [w337]
                        tunnel: w333 -> [w350] mode=indexing
                        tunnel: w332 -> [w349] mode=indexing
                        tunnel: w331 -> [w348]
                        tunnel: w330 -> [w347]
                        tunnel: w329 -> [w346]
                        tunnel: [w345] -> w328 mode=indexing
                        tunnel: w327 -> [w344]
                        tunnel: w326 -> [w343]
                        tunnel: w325 -> [w342]
                        tunnel: w324 -> [w341]
                        tunnel: w323 -> [w340]
                        tunnel: [w339] -> w322
                        tunnel: w321 -> [w336]
                        tunnel: w320 -> [w335]
                        i -> [w338]
                        n91 = stacked-sequence {
                          seq-local: [w356 _] -> [_ w375]
                          seq-local: [w352 _] -> [_ w374]
                          tunnel: w350 -> [w365 _]
                          tunnel: w349 -> [w364 _]
                          tunnel: w348 -> [w363 _]
                          tunnel: w347 -> [w362 _]
                          tunnel: w346 -> [w360 _]
                          tunnel: [w359 _] -> w345
                          tunnel: w344 -> [_ w377]
                          tunnel: w343 -> [_ w376]
                          tunnel: w342 -> [_ _]
                          tunnel: w338 -> [w358 _]
                          tunnel: w341 -> [w354 _]
                          tunnel: w340 -> [w353 _]
                          tunnel: [_ w373] -> w339
                          tunnel: w338 -> [_ _]
                          tunnel: w337 -> [_ _]
                          tunnel: w336 -> [w351 _]
                          tunnel: w335 -> [_ w370]
                          frame #0 {
                            n92 = Equal To 0?(x=w358) -> (x = 0?=w357:bool)
                            n93 = call "zern2command_test.vi"("Initial haso file"=w362, "error in (no error)"=w353, "interaction matrix file"=w363, "Zern coef in"=w364, "Zern index in"=w365) -> ("error out"=w352:errorcluster, "Zern coef out"=w355:sgl[], "Offset positions"=w361:sgl[])  [unwired: 4 in]
                            n94 = case shown="False" w357 {
                              tunnel: [w366 w367] -> w356
                              tunnel: w355 -> [w366 _]
                              tunnel: w354 -> [_ _]
                              tunnel: w351 -> [_ w367]
                              frame False {
                              }
                              frame True {
                              }
                            }
                            n95 = Add(x=w360, y=w361) -> (x+y=w359:dbl[])
                          }
                          frame #1 {
                            n96 = Number To Fractional String(number=w370, precision (6)=0) -> (F-format string=w369:string)  [unwired: 2 in]
                            n97 = Concatenate Strings(w377, w376, "_", w369, "_coeff.txt") -> (w385:string)
                            n98 = String To Path(string=w385) -> (path=w384:path)
                            n99 = Open/Create/Replace File(file path (use dialog)=w384, error in=w374, operation (0:open)=3) -> (refnum out=w381:refnum<file>, error out=w382:errorcluster)  [unwired: 3 in, 1 out]
                            n100 = Array To Spreadsheet String(array=w375, 3:"%f") -> (spreadsheet string=w372:string)  [unwired: 1 in]
                            n101 = Set File Position(refnum=w381, from (0:start)=1, error in=w382) -> (refnum out=w379:refnum<file>, error out=w378:errorcluster)  [unwired: 1 in]
                            n102 = Write to Text File(file (use dialog)=w379, text=w372, error in=w378) -> (error out=w373:errorcluster)  [unwired: 1 in, 2 out]
                          }
                        }
                      }
                    }
                    frame #2 {
                      n103 = Number To Fractional String(number=w389, precision (6)=0) -> (F-format string=w388:string)  [unwired: 2 in]
                      n104 = Concatenate Strings(w394, w393, "_", w388, "_IniAbr+offset.txt") -> (w404:string)
                      n105 = String To Path(string=w404) -> (path=w402:path)
                      n106 = Open/Create/Replace File(file path (use dialog)=w402, error in=w392, operation (0:open)=3) -> (refnum out=w399:refnum<file>, error out=w400:errorcluster)  [unwired: 3 in, 1 out]
                      n107 = Array To Spreadsheet String(array=w395, 3:"%f") -> (spreadsheet string=w406:string)  [unwired: 1 in]
                      n108 = Set File Position(refnum=w399, from (0:start)=1, error in=w400) -> (refnum out=w397:refnum<file>, error out=w396:errorcluster)  [unwired: 1 in]
                      n109 = Write to Text File(file (use dialog)=w397, text=w406, error in=w396) -> (error out=w391:errorcluster)  [unwired: 1 in, 2 out]
                    }
                  }
                }
                frame #6 {
                  # "set andor kinetics and spooling, \nstart acquire and wait for the external trigger"
                  n110 = Number To Fractional String(number=w408, precision (6)=0) -> (F-format string=w409:string)  [unwired: 2 in]
                  n111 = Concatenate Strings(w414, w413, "_PhsDiv_ToBeDeleted_", w409) -> (w411:string)
                  n112 = call "SetSpool_WaitForExtTrigger.vi"("path and name"=w411, "Kinetic Series"=w415) -> ()  [unwired: 10 in]
                }
                frame #7 {
                  # "take phase diversity pictures"
                  n113 = for {
                    N: w422 -> [_]
                    tunnel: w427 -> [w438]
                    tunnel: w426 -> [w437]
                    tunnel: w425 -> [w436]
                    tunnel: w421 -> [w435]
                    tunnel: w424 -> [w434]
                    tunnel: w423 -> [w433] mode=indexing
                    tunnel: w420 -> [w432]
                    tunnel: w419 -> [w431]
                    tunnel: [w430] -> w417
                    tunnel: [w429] -> w418
                    tunnel: w416 -> [w428]
                    n114 = stacked-sequence {
                      seq-local: [w439 _] -> [_ w448]
                      tunnel: w438 -> [_ w450]
                      tunnel: w437 -> [_ _]
                      tunnel: w436 -> [_ _]
                      tunnel: w435 -> [_ _]
                      tunnel: w434 -> [_ _]
                      tunnel: w433 -> [w440 _]
                      tunnel: w432 -> [_ w449]
                      tunnel: w431 -> [w441 _]
                      tunnel: [_ w447] -> w430
                      tunnel: [_ w446] -> w429
                      tunnel: w428 -> [w442 _]
                      frame #0 {
                        # "response time of mirror"
                        n115 = call <userlib>:"LVClass_WavefrontCorrector Move to Absolute Position.vi"("WavefrontCorrector in"=w442, "Absolute Positions"=w440, "error in (no error)"=w441) -> ("error out"=w439:errorcluster)  [unwired: 11 in, 1 out]
                        n116 = Add(x=5, y=10) -> (x+y=w443:i32)
                        n117 = Wait (ms)(milliseconds to wait=w443) -> ()  [unwired: 1 out]
                      }
                      frame #1 {
                        n118 = for {
                          N: w450 -> [_]
                          tunnel: w449 -> [w455]
                          tunnel: w448 -> [w453]
                          tunnel: [w452] -> w447
                          tunnel: [w451] -> w446
                          n119 = local read "EMCCD trigger port"() -> (w458:tag)
                          n120 = Add(x=w455, y=0.04) -> (x+y=w454:dbl)
                          n121 = Multiply(x=w454, y=1000.0) -> (x*y=w451:dbl)
                          n122 = call "trig EMCCD.vi"("error in (no error)"=w453, "exp time (ms)"=w451, "lines"=w458) -> ("error out"=w452:errorcluster)
                        }
                      }
                    }
                  }
                }
                frame #8 {
                  # "send out a trigger to EMCCD to end the aquisition."
                  n123 = local read "EMCCD trigger port"() -> (w460:tag)
                  n124 = call "trig EMCCD.vi"("exp time (ms)"=w459, "lines"=w460) -> ()  [unwired: 1 in, 1 out]
                }
                frame #9 {
                  w468 = 0
                  # "save phase diversity pictures:\npictures per phase*number of phases (Eg: 2*5=10 pictures in this file)"
                  n125 = Number To Fractional String(number=w461, precision (6)=w468) -> (F-format string=w467:string)  [unwired: 2 in]
                  n126 = Concatenate Strings(w472, "_", w467) -> (w463:string)
                  "phase diversity file name" <- w463
                  n127 = Concatenate Strings(w463, ".tif") -> (w464:string)
                  n128 = Concatenate Strings(w471, w464) -> (w466:string)
                  n129 = call <userlib>:"SaveAsTiff.vi"("path"=w466, "palette"="C:\\Program Files\\Andor SOLIS\\GREY.PAL", "position"=w468, "type"=1) -> ()  [unwired: 10 in, 2 out]
                }
                frame #10 {
                  # "run matlab correction?"
                  n130 = case shown="True" w482 {
                    tunnel: w488 -> [_ w505]
                    tunnel: w489 -> [_ w504]
                    tunnel: w487 -> [_ w503]
                    tunnel: w486 -> [_ w502]
                    tunnel: w484 -> [_ w501]
                    tunnel: w485 -> [_ w500]
                    tunnel: w483 -> [_ w499]
                    tunnel: w475 -> [_ w498]
                    tunnel: w481 -> [_ _]
                    tunnel: [0 w497] -> w474
                    tunnel: w480 -> [_ w496]
                    tunnel: [errorcluster {"status"=FALSE, "code"=0, "source"=""} ("Error out 2") w495] -> w479
                    tunnel: w478 -> [_ w494]
                    tunnel: w477 -> [_ w493]
                    tunnel: w476 -> [_ _]
                    tunnel: w473 -> [_ w492]
                    frame False {
                    }
                    frame True {
                      # "matlab reconstructed Zern"
                      n131 = stacked-sequence {
                        seq-local: [w523 _ _ _ _ _ _ _ _ _ _] -> [_ _ _ _ _ _ w578 _ _ _ _]
                        seq-local: [w529 _ _ _ _ _ _ _ _ _ _] -> [_ _ _ _ _ _ w574 _ _ _ _]
                        seq-local: [_ _ _ _ w556 _ _ _ _ _ _] -> [_ _ _ _ _ w563 _ _ _ _ _]
                        seq-local: [_ _ w544 _ _ _ _ _ _ _ _] -> [_ _ _ w551 _ _ _ _ _ _ _]
                        seq-local: [_ _ _ w553 _ _ _ _ _ _ _] -> [_ _ _ _ w557 _ _ _ _ _ _]
                        seq-local: [_ w536 _ _ _ _ _ _ _ _ _] -> [_ _ _ _ _ _ _ _ _ _ w605]
                        seq-local: [_ _ _ _ _ _ w567 _ _ _ _] -> [_ _ _ _ _ _ _ w583 _ _ _]
                        tunnel: w505 -> [w528 w539 _ _ _ _ _ _ _ w594 _]
                        tunnel: w504 -> [w522 w538 _ _ _ _ _ _ _ w593 _]
                        tunnel: w503 -> [_ _ _ _ _ _ w577 _ _ _ _]
                        tunnel: w502 -> [_ _ _ _ w558 _ w576 _ _ _ _]
                        tunnel: w501 -> [_ _ _ w555 _ w565 _ w585 w591 _ _]
                        tunnel: w499 -> [_ _ w545 _ _ _ _ _ _ _ _]
                        tunnel: [_ _ _ w554 _ _ _ _ _ _ _] -> _
                        tunnel: w500 -> [_ _ _ w554 _ _ _ w584 _ _ _]
                        tunnel: w498 -> [w520 w537 _ _ _ _ _ _ _ w595 _]
                        tunnel: [w507 _ _ _ _ _ _ _ _ _ _] -> w497
                        tunnel: w496 -> [_ _ w546 _ _ _ _ _ _ _ _]
                        tunnel: [_ _ _ _ _ _ _ w582 _ _ _] -> w495
                        tunnel: w494 -> [_ _ w547 _ w559 _ w570 _ _ _ _]
                        tunnel: w493 -> [_ w540 _ _ _ _ _ _ _ _ w603]
                        tunnel: w492 -> [_ _ _ _ _ _ w566 _ _ _ _]
                        frame #0 {
                          # "MATLAB does the reconstruction, written by Min Guo"
                          # "other parameters are default in this VI"
                          n132 = Number To Fractional String(number=w520, precision (6)=0) -> (F-format string=w518:string)  [unwired: 2 in]
                          n133 = Concatenate Strings(w522, "_", w518) -> (w506:string)
                          n134 = String To Path(string=w528) -> (path=w530:path)
                          n135 = Concatenate Strings(w528, w506) -> (w527:string)
                          n136 = String To Path(string=w527) -> (path=w526:path)
                          n137 = call "recon_zern_fileIO_MATLAB.vi"("Number of Phase"="Number of Phase", "Number for average"="Number for average", "Crop Size of image"="Crop Size of image", "Background Value"="Background Value", "Zernike Order"="Zernike Order", "Use GPU"="Use GPU", "Iteration Number"="Iteration Number", "File Name"=w506, "Gamma Value"="Gamma Value", "Path In"=w530, "Show Input"="Show Input", "Path Out"=w526, "Show Recon"="Show Recon") -> ("Zern coef out"=w524:sgl[], "RMSE Value"=w507:dbl, "error out"=w529:errorcluster)  [unwired: 3 in, 1 out]
                          n138 = case shown="False" "Keep Reconstructed Defocus component?" {
                            tunnel: w524 -> [w531 w535]
                            tunnel: [w531 w532] -> w523
                            frame False {
                            }
                            frame True {
                              n139 = Replace Array Subset(array=w535, new element=0.0, index=2) -> (w532:sgl[])
                            }
                          }
                        }
                        frame #1 {
                          # "set andor kinetics and spooling, \nstart acquire and wait for the external trigger"
                          n140 = Number To Fractional String(number=w537, precision (6)=0) -> (F-format string=w541:string)  [unwired: 2 in]
                          n141 = Concatenate Strings(w539, w538, "_Corr_ToBeDeleted_", w541) -> (w536:string)
                          n142 = call "SetSpool_WaitForExtTrigger.vi"("path and name"=w536, "Kinetic Series"=w540) -> ()  [unwired: 10 in]
                        }
                        frame #2 {
                          # "groundtruth command"
                          # "response time of mirror"
                          n143 = call <userlib>:"LVClass_WavefrontCorrector Move to Absolute Position.vi"("WavefrontCorrector in"=w547, "Absolute Positions"=w546, "error in (no error)"=w545) -> ("error out"=w544:errorcluster)  [unwired: 11 in, 1 out]
                          n144 = Add(x=5, y=10) -> (x+y=w548:i32)
                          n145 = Wait (ms)(milliseconds to wait=w548) -> ()  [unwired: 1 out]
                        }
                        frame #3 {
                          # "take offset/groundtruth picture, only one"
                          n146 = local read "EMCCD trigger port"() -> (w552:tag)
                          n147 = call "trig EMCCD.vi"("error in (no error)"=w551, "exp time (ms)"=w555, "lines"=w552) -> ("error out"=w553:errorcluster)
                        }
                        frame #4 {
                          # "aberrated picture command"
                          # "response time of mirror"
                          n148 = call <userlib>:"LVClass_WavefrontCorrector Move to Absolute Position.vi"("WavefrontCorrector in"=w559, "Absolute Positions"=w558, "error in (no error)"=w557) -> ("error out"=w556:errorcluster)  [unwired: 11 in, 1 out]
                          n149 = Add(x=5, y=10) -> (x+y=w560:i32)
                          n150 = Wait (ms)(milliseconds to wait=w560) -> ()  [unwired: 1 out]
                        }
                        frame #5 {
                          # "take offset+initial aberr picture, only one"
                          n151 = local read "EMCCD trigger port"() -> (w564:tag)
                          n152 = call "trig EMCCD.vi"("error in (no error)"=w563, "exp time (ms)"=w565, "lines"=w564) -> ()  [unwired: 1 out]
                        }
                        frame #6 {
                          w581 = 1
                          # "correction command"
                          # "response time of mirror"
                          n153 = call-poly <vilib>:"Ramp Pattern.vi"("start"=w581, "end"=32, "delta"=w581) -> ("Ramp Pattern"=w579:dbl[])  [unwired: 6 in, 2 out]
                          n154 = call "zern2command_test.vi"("Initial haso file"=w566, "error in (no error)"=w574, "interaction matrix file"=w577, "Zern coef in"=w578, "Zern index in"=w579) -> ("error out"=w568:errorcluster, "Offset positions"=w575:sgl[])  [unwired: 4 in, 1 out]
                          n155 = Add(x=w576, y=w575) -> (x+y=w569:dbl[])
                          n156 = call <userlib>:"LVClass_WavefrontCorrector Move to Absolute Position.vi"("WavefrontCorrector in"=w570, "Absolute Positions"=w569, "error in (no error)"=w568) -> ("error out"=w567:errorcluster)  [unwired: 11 in, 1 out]
                          n157 = Add(x=5, y=10) -> (x+y=w571:i32)
                          n158 = Wait (ms)(milliseconds to wait=w571) -> ()  [unwired: 1 out]
                        }
                        frame #7 {
                          # "corrected pictures"
                          n159 = for {
                            N: w584 -> [_]
                            tunnel: w585 -> [w588]
                            shift-right: [w586] -> w582
                            shift-left: w583 -> [w587]
                            n160 = local read "EMCCD trigger port"() -> (w589:tag)
                            n161 = call "trig EMCCD.vi"("error in (no error)"=w587, "exp time (ms)"=w588, "lines"=w589) -> ("error out"=w586:errorcluster)
                          }
                        }
                        frame #8 {
                          # "one more trigger to end picture acquisition"
                          n162 = local read "EMCCD trigger port"() -> (w590:tag)
                          n163 = call "trig EMCCD.vi"("exp time (ms)"=w591, "lines"=w590) -> ()  [unwired: 1 in, 1 out]
                        }
                        frame #9 {
                          w598 = 0
                          # "save:\none groundtruth picture\none offset+abrr picture\nPictures per phase*corrected picture"
                          n164 = Number To Fractional String(number=w595, precision (6)=w598) -> (F-format string=w597:string)  [unwired: 2 in]
                          n165 = Concatenate Strings(w593, "_grdtrth_abrr_Corr_", w597, ".tif") -> (w602:string)
                          "Corrected Picture name" <- w602
                          n166 = Concatenate Strings(w594, w602) -> (w596:string)
                          n167 = call <userlib>:"SaveAsTiff.vi"("path"=w596, "palette"="C:\\Program Files\\Andor SOLIS\\GREY.PAL", "position"=w598, "type"=1) -> ()  [unwired: 10 in, 2 out]
                        }
                        frame #10 {
                          n168 = case shown="True" TRUE {
                            tunnel: w605 -> [_ w607]
                            tunnel: w603 -> [_ w606]
                            frame False {
                            }
                            frame True {
                              # "delete spooling data"
                              n169 = for {
                                N: w606 -> [_]
                                tunnel: w607 -> [w614]
                                i -> [w612]
                                n170 = Number To Fractional String(number=w612, precision (6)=0) -> (F-format string=w610:string)  [unwired: 2 in]
                                n171 = Concatenate Strings(w614, "000000000", w610, ".dat") -> (w609:string)
                                n172 = String To Path(string=w609) -> (path=w615:path)
                                n173 = Delete(path (use dialog)=w615) -> ()  [unwired: 4 in, 3 out]
                              }
                            }
                          }
                        }
                      }
                    }
                  }
                }
                frame #11 {
                  # "delete spooling data of phase diversity"
                  n174 = case shown="True" TRUE {
                    tunnel: w618 -> [_ w620]
                    tunnel: w616 -> [_ w619]
                    frame False {
                    }
                    frame True {
                      n175 = for {
                        N: w619 -> [_]
                        tunnel: w620 -> [w629]
                        i -> [w622]
                        n176 = Number To Decimal String(number=w622) -> (decimal integer string=w627:string)  [unwired: 1 in]
                        n177 = String Length(string=w627) -> (length=w625:i32)
                        n178 = Subtract(x=10, y=w625) -> (x-y=w624:i32)
                        n179 = for {
                          N: w624 -> [_]
                          shift-right: [w636] -> w621
                          shift-left: "" -> [w635]
                          n180 = Concatenate Strings(w635, "0") -> (w636:string)
                        }
                        n181 = Number To Fractional String(number=w622, precision (6)=0) -> (F-format string=w631:string)  [unwired: 2 in]
                        n182 = Concatenate Strings(w629, w621, w631, ".dat") -> (w628:string)
                        n183 = String To Path(string=w628) -> (path=w633:path)
                        n184 = Delete(path (use dialog)=w633) -> ()  [unwired: 4 in, 3 out]
                      }
                    }
                  }
                }
              }
            }
          }
          frame #2 {
            # "shut down shutter of 488nm laser"
            n185 = invoke class="MG17Motor" method="SC_Disable"(reference=w640, "lChanID"=w639) -> (reference out=w638:refnum<k7>, "lChanID"=w637:i32)  [unwired: 2 in, 2 out]
          }
          frame #3 {
            n186 = Concatenate Strings(w642, w641, "_RMSE.txt") -> (w648:string)
            n187 = String To Path(string=w648) -> (path=w647:path)
            n188 = Number To Fractional String(number=w644) -> (F-format string=w645:string[])  [unwired: 3 in]
            n189 = Write to Text File(file (use dialog)=w647, text=w645) -> (error out=w643:errorcluster)  [unwired: 2 in, 2 out]
          }
        }
        n190 = Merge Errors(w180, w179, w175) -> (w174:errorcluster)
        "Error out" <- w174
        n191 = Unbundle(w174) -> ("status"=w170:bool)  [unwired: 2 out]
        n192 = case shown="True" w170 {
          tunnel: [w195 w196] -> w173
          tunnel: w170 -> [w194 w196]
          frame False {
            n193 = Not(x=w194) -> (.not. x?=w195:bool)
          }
          frame True {
          }
        }
        n194 = Or(x=w173, y="?") -> (x .or. y?=w171:bool)
      }
    }
    frame #4 {
      n195 = case shown="True" "Turn off EMCCD when finished?" {
        frame False {
        }
        frame True {
          n196 = flat-sequence {
            frame #0 {
              n197 = call <userlib>:"CoolerOFF.vi"() -> ()  [unwired: 2 in, 2 out]
            }
            frame #1 {
              # "shut down EMCCD"
              n198 = call <userlib>:"ShutDown.vi"() -> ()  [unwired: 2 in, 2 out]
            }
          }
        }
      }
    }
    frame #5 {
      # "shut down casao"
      n199 = call <userlib>:"LVClass_WavefrontCorrector dtor.vi"("WavefrontCorrector in"=w653, "error in (no error)"=w651) -> ("error out"=w650:errorcluster)  [unwired: 12 in, 1 out]
      n200 = call <userlib>:"LVClass_WavefrontCorrectorSet dtor.vi"("WavefrontCorrectorSet in"=w652, "error in (no error)"=w650) -> ()  [unwired: 12 in, 2 out]
      n201 = invoke class="MG17Motor" method="StopCtrl"(reference=w654) -> ()  [unwired: 2 in, 3 out]
    }
  }
